vi "Test multiplexeur.vi"() -> ()   [LabVIEW 2018]
panel:
  out "Graphe déroulant":dynamicdata(graph)
  out "Numérique":i32
  in  "stop":bool
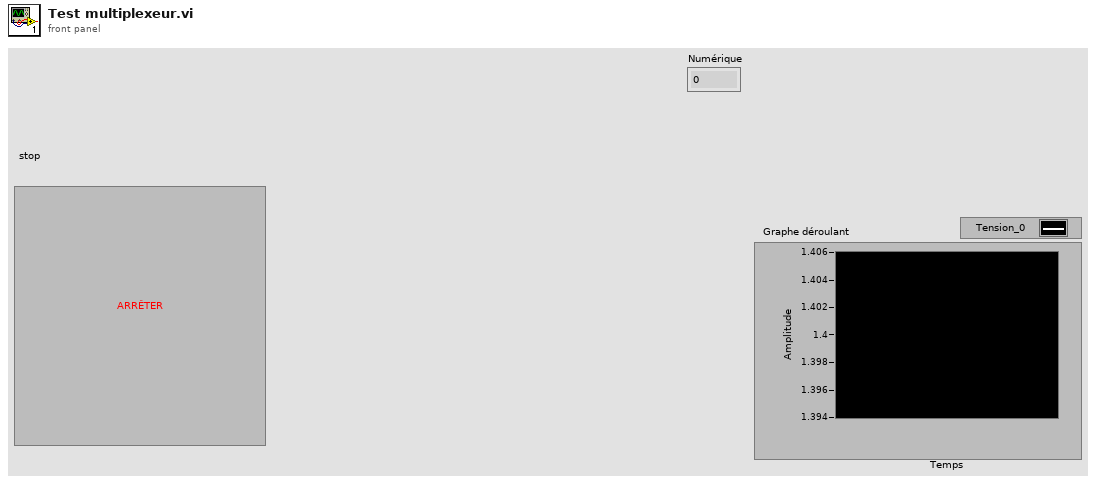
[diagram p1: front panel]
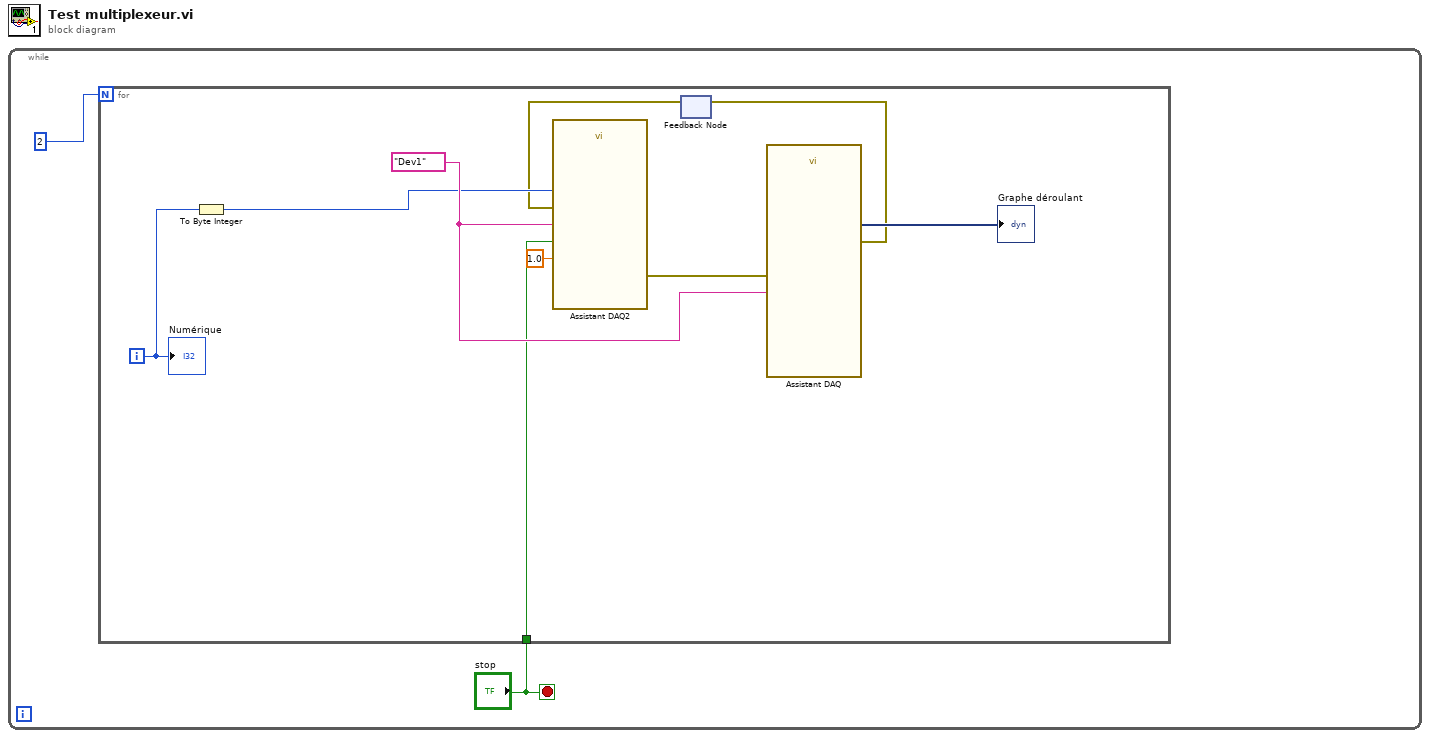
[diagram p0: block diagram]
diagram:
  n1 = while {
    stop <- "stop" stop-if-true
    n2 = for {
      N: 2 -> [_]
      tunnel: "stop" -> [w5]
      i -> [w8]
      w10 = tag "Dev1" ("nom du périphérique")
      n3 = To Byte Integer(number=w8) -> (8bit integer=w7:i8)
      n4 = feedback #1() -> (w3:errorcluster)  [unwired: 1 in]
      n5 = call "Assistant DAQ2"("data"=w7, "timeout (s)"=1.0, "error in"=w3, "stop (T)"=w5, "nom du périphérique"=w10) -> ("error out"=w11:errorcluster)  [unwired: 13 in, 1 out]
      n6 = call "Assistant DAQ"("error in"=w11, "nom du périphérique"=w10) -> ("data"=→"Graphe déroulant":dynamicdata, "error out"=w4:errorcluster)  [unwired: 15 in, 1 out]
      n7 = feedback-in #1(w4) -> ()
      "Numérique" <- w8
    }
  }
